vi "getAvailableCount.vi"(8 "error in (no error)":errorcluster, 11 "IReader in":refnum<class "IReader.lvclass">) -> (0 "error out":errorcluster, 2 "Available Count":i32, 3 "IReader out":refnum<class "IReader.lvclass">)   [LabVIEW 2022 SP3, in "openDAQ.lvlib" / "IBaseObject.lvlib" / "IReader.lvlib" / "IReader.lvclass"]
uses:
  <instrlib>/openDAQ/Public/Classes/IReader/IReader.lvclass
  C:/Program Files (x86)/National Instruments/LabVIEW 2022/instr.lib/openDAQ/Public/Classes/IBaseObject/IBaseObject.lvclass
  <instrlib>/openDAQ/Public/Classes/IBaseObject/IBaseObject.lvclass/IBaseObject.ctl
  <instrlib>/openDAQ/Public/Classes/IBaseObject/Accessor/Read reference.vi
  <instrlib>/openDAQ/Public/Classes/IBaseObject/Accessor/Write reference.vi
  <instrlib>/openDAQ/Binaries/Windows/x86/copendaq32.dll
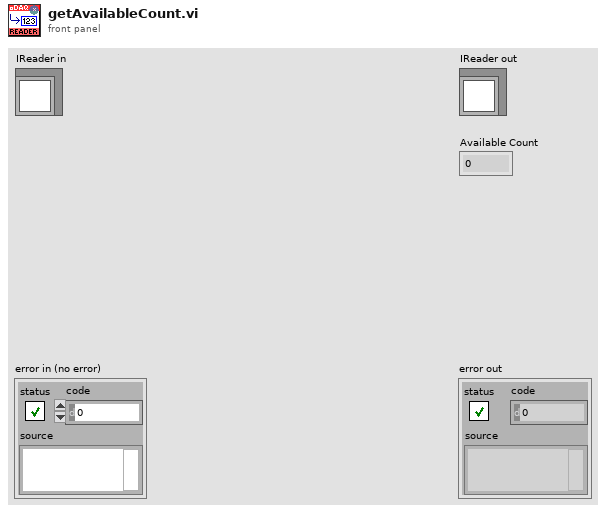
[diagram p1: front panel]
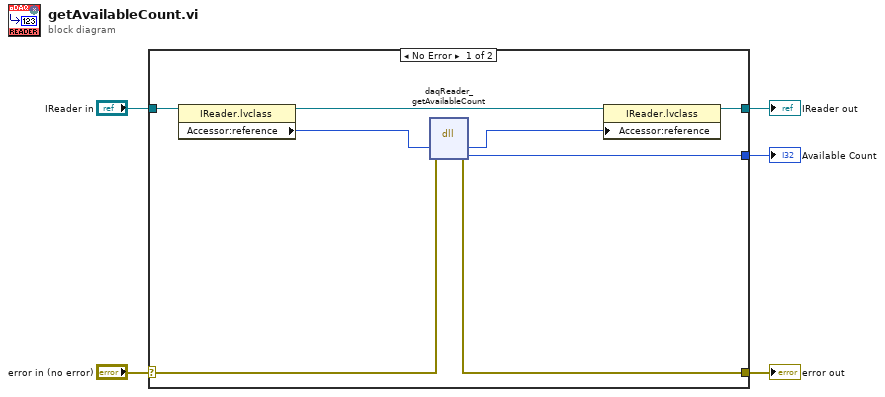
[diagram p0: block diagram]
diagram:
  n1 = case shown="No Error" "error in (no error)" {
    selector: "error in (no error)" -> [w12 w15]
    tunnel: [w11 w15] -> w4
    tunnel: [w9 w14] -> w2
    tunnel: "IReader in" -> [w13 w14]
    tunnel: [w6 _] -> w1
    frame No Error {
      n2 = property class="IReader.lvclass"(reference=w13) -> (reference out=w10:refnum<class "IReader.lvclass">, "Accessor:reference"=w8:i64)  [unwired: 1 in, 1 out]
      n3 = dll-call lib="C:/Program Files (x86)/National Instruments/LabVIEW 2022/instr.lib/openDAQ/Binaries/Windows/x86/copendaq*.*" fn="daqReader_getAvailableCount"(error in=w12, "reader"=w8) -> (error out=w11:errorcluster, "reader"=w7:i64, "availableCount"=w6:i32)  [unwired: 4 in, 1 out]
      n4 = property class="IReader.lvclass"(reference=w10, "Accessor:reference"=w7) -> (reference out=w9:refnum<class "IReader.lvclass">)  [unwired: 1 in, 1 out]
    }
    frame Error {
    }
  }
  "error out" <- w4
  "IReader out" <- w2
  "Available Count" <- w1
